vi "selectFiles.vi"(8 "error in (no error)":errorcluster, 11 "FileSelector in":refnum<class "FileSelector.lvclass">) -> (0 "error out":errorcluster, 1 "cancelledIsTrue":bool caption="cancelled", 2 "selected paths":path[](array[path]), 3 "FileSelector out":refnum<class "FileSelector.lvclass">)   [LabVIEW 2016, in "FileSelector.lvclass"]
uses:
  FileSelector.lvclass
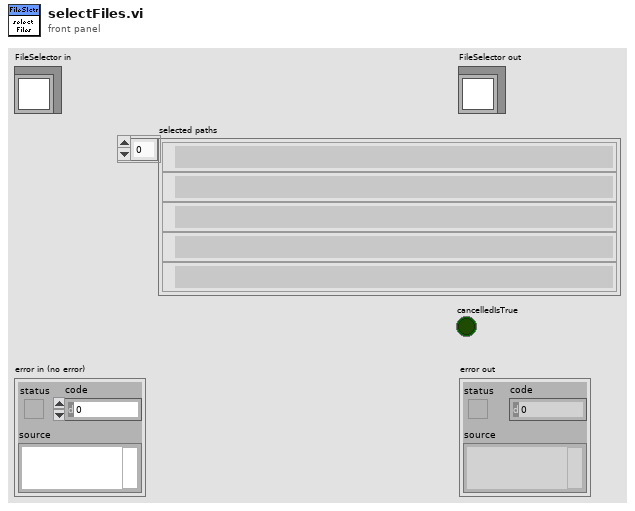
[diagram p1: front panel]
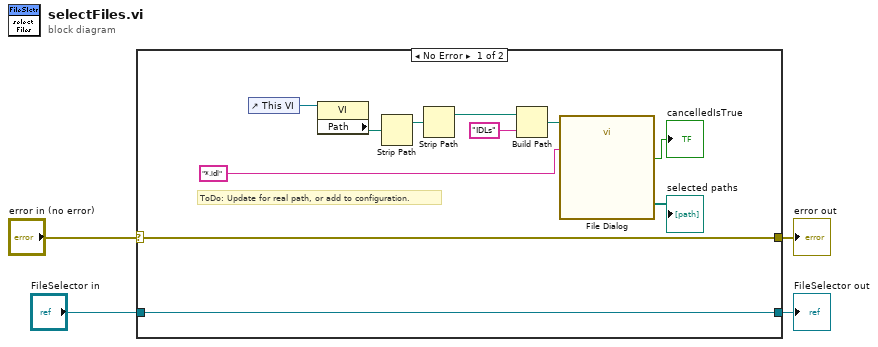
[diagram p0: block diagram]
diagram:
  n1 = case shown="No Error" "error in (no error)" {
    selector: "error in (no error)" -> [w14 w17]
    tunnel: [w14 w17] -> w3
    tunnel: [w15 w16] -> w1
    tunnel: "FileSelector in" -> [w15 w16]
    frame No Error {
      # "ToDo: Update for real path, or add to configuration."
      n2 = control-ref of="This VI"() -> (w13:refnum<vi>)
      n3 = property class="VI"(reference=w13) -> ("Path"=w12:path)  [unwired: 1 in, 2 out]
      n4 = Strip Path(path=w12) -> (stripped path=w7:path)  [unwired: 1 out]
      n5 = Strip Path(path=w7) -> (stripped path=w6:path)  [unwired: 1 out]
      n6 = Build Path(base path=w6, name or relative path="IDLs") -> (appended path=w10:path)
      n7 = call "File Dialog"("start path"=w10, "pattern (all files)"="*.idl") -> ("selected paths"=→"selected paths":path[], "cancelled"=→"cancelledIsTrue":bool)  [unwired: 10 in, 2 out]
    }
    frame Error {
    }
  }
  "error out" <- w3
  "FileSelector out" <- w1
